vi "kissia_rasPico Module.vi"(5 "Enable":bool=TRUE, 6 "Timeout(s)":dbl=2.0, 7 "Command":T1, 8 "error in (no error)":errorcluster, 10 "VALVE":bool, 11 "VISA resource name":refnum<visa-resource-name>="COM39") -> (0 "error out":errorcluster, 2 "read string":string, 3 "TimeOut":bool, 4 "write string":string)   [LabVIEW 2017]
uses:
  kissia_rasPico Module.ctl
  kissia_ArduinoMicro Module.ctl
  <vilib>/Instr/_visa.llb/VISA Configure Serial Port (Instr).vi
panel:
  out "Bytes at Serial Port":u32
  # "Output Data"
  # "Input Data"
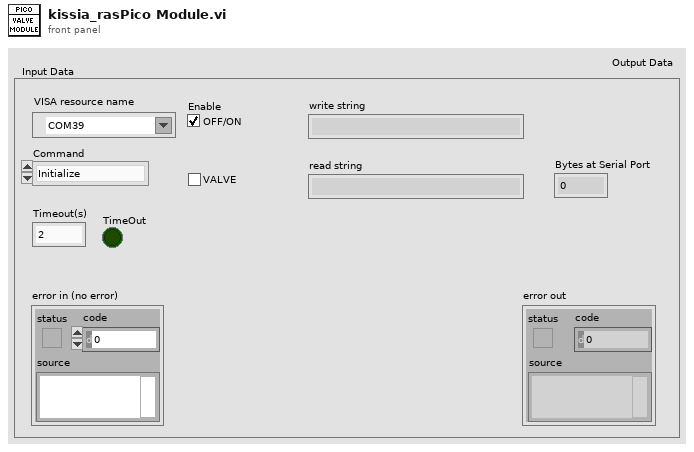
[diagram p1: front panel]
types:
  T1 = typedef "kissia_rasPico Module.ctl" = enum16{"Initialize", "Read Data", "Write Data", "Enable", "Disable", "Shutdown"}
  T2 = typedef "kissia_ArduinoMicro Module.ctl" = enum16{"Initialize", "Read Data", "Write Data", "Enable", "Disable", "Shutdown"}
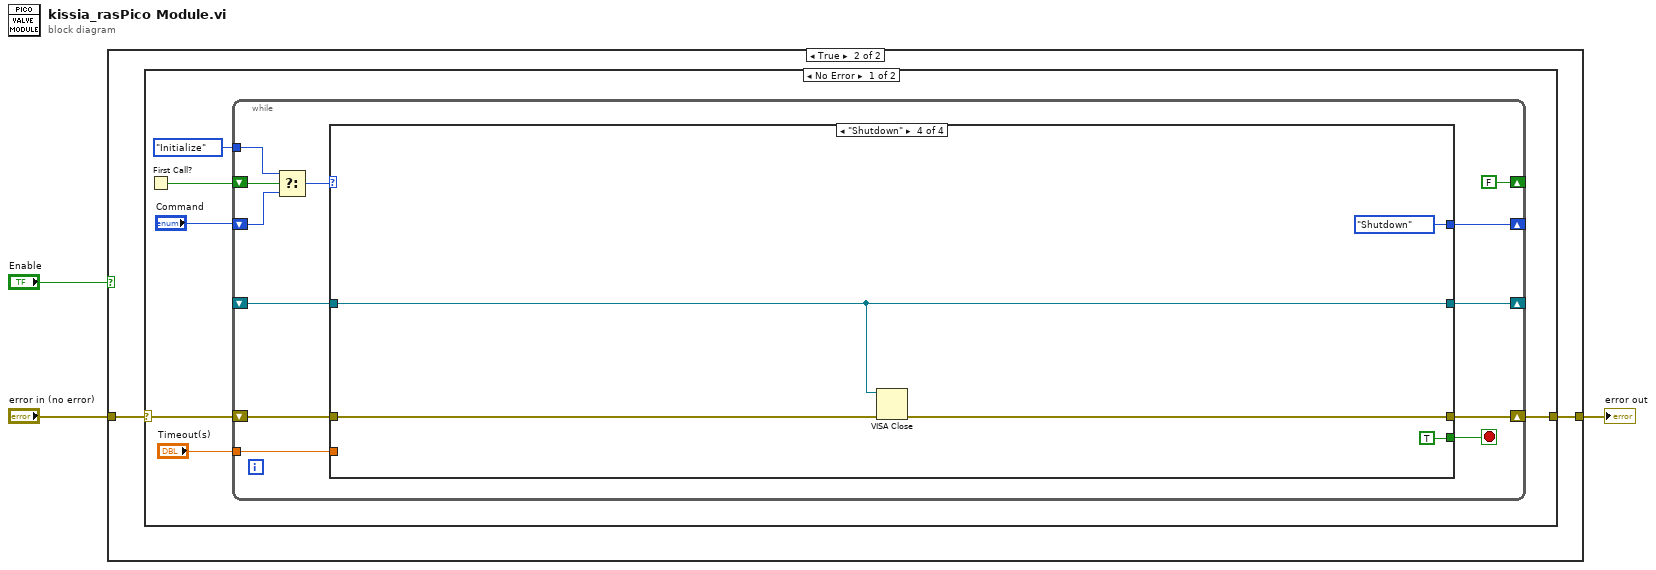
[diagram p0: block diagram]
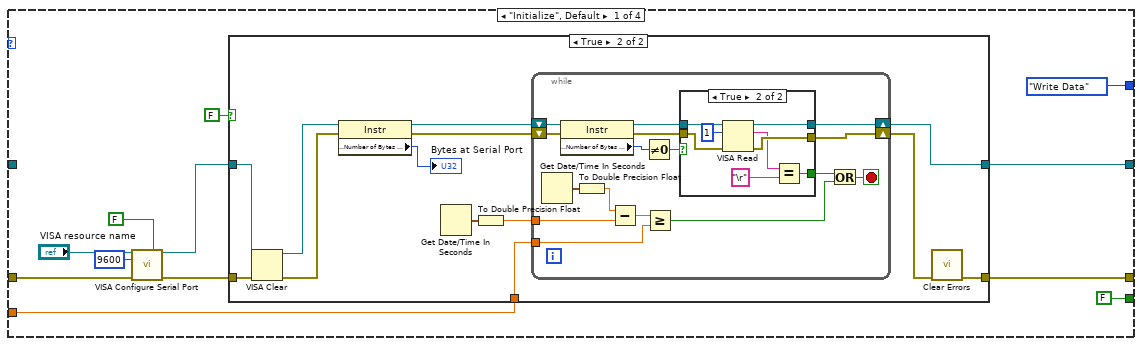
[diagram p3: hidden frame]
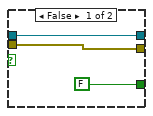
[diagram p5: hidden frame]
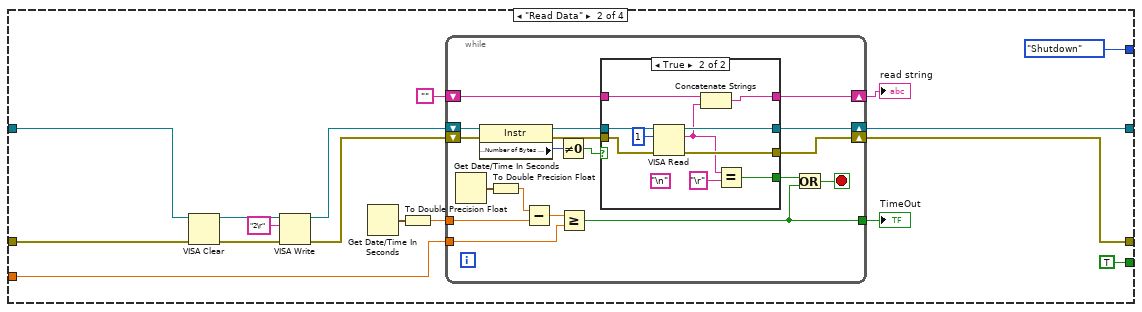
[diagram p6: hidden frame]
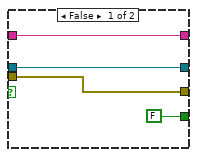
[diagram p7: hidden frame]
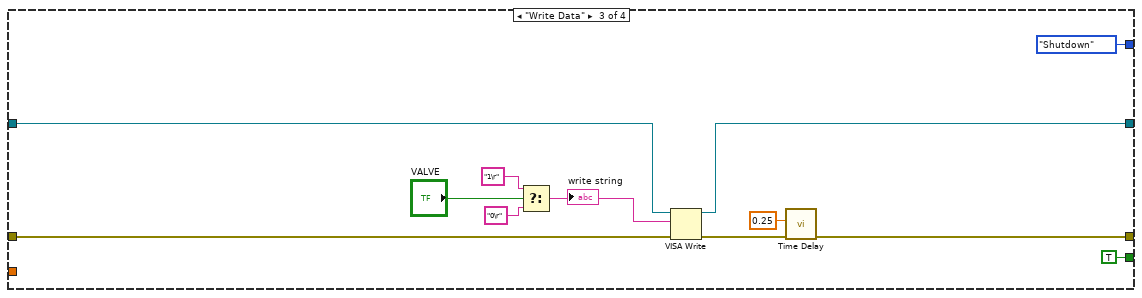
[diagram p8: hidden frame]
diagram:
  n1 = case shown="True" "Enable" {
    tunnel: "error in (no error)" -> [w4 w6]
    tunnel: [w4 w5] -> w2
    frame False {
    }
    frame True {
      n2 = case shown="No Error" w6 {
        selector: w6 -> [w10 w145]
        tunnel: [w9 w145] -> w5
        frame No Error {
          n3 = First Call?() -> (First Call?: T/F=w12:bool)
          n4 = while {
            shift-right: [w15] -> _
            shift-left: "Command" -> [w21]
            shift-right: [w18] -> w9
            shift-left: w10 -> [w19]
            shift-right: [FALSE ("First Call?: T/F")] -> _
            shift-left: w12 -> [w24]
            tunnel: kissia_ArduinoMicro_Module."Initialize" ("t") -> [w23]
            shift-right: [w17] -> _
            shift-left: _ -> [w16]
            tunnel: "Timeout(s)" -> [w13]
            stop <- w14 stop-if-true
            n5 = Select(t=w23, s=w24, f=w21) -> (s? t:f=w20:T2)
            n6 = case shown="\"Shutdown\"" w20 {
              tunnel: w19 -> [w31 w86 w139 w141]
              tunnel: [w26 w87 w133 w140] -> w18
              tunnel: [w30 w88 w136 w142] -> w17
              tunnel: w16 -> [_ w85 w132 w142]
              tunnel: [kissia_ArduinoMicro_Module."Write Data" ("t") kissia_ArduinoMicro_Module."Shutdown" ("t") kissia_ArduinoMicro_Module."Shutdown" ("t") kissia_ArduinoMicro_Module."Shutdown" ("t")] -> w15
              tunnel: [FALSE ("Enable Termination\nChar (T)") TRUE ("Enable Termination\nChar (T)") TRUE ("Enable Termination\nChar (T)") TRUE ("Enable Termination\nChar (T)")] -> w14
              tunnel: w13 -> [w29 w91 _ _]
              frame "Initialize", Default {
                n7 = call-poly "VISA Configure Serial Port"("VISA resource name"="VISA resource name", "Enable Termination\nChar (T)"=FALSE ("Enable Termination\nChar (T)"), "baud rate (9600)"=u32 9600, "error in (no error)"=w31) -> ("VISA resource name out"=w28:refnum<visa-resource-name>, "error out"=w27:errorcluster)  [unwired: 10 in]
                n8 = case shown="True" FALSE {
                  tunnel: [w38 w48] -> w30
                  tunnel: w29 -> [_ w47]
                  tunnel: w28 -> [w38 w46]
                  tunnel: w27 -> [w37 w45]
                  tunnel: [w37 w43] -> w26
                  frame False {
                  }
                  frame True {
                    n9 = VISA Clear(VISA resource name=w46, error in (no error)=w45) -> (VISA resource name out=w40:refnum<visa-resource-name>, error out=w42:errorcluster)
                    n10 = property class="Instr"(reference=w40, error in=w42) -> (reference out=w39:refnum<visa-resource-name>, error out=w41:errorcluster, "Serial Settings:Number of Bytes at Serial Port"=→"Bytes at Serial Port":u32)
                    n11 = Get Date/Time In Seconds() -> (seconds since 1Jan1904=w51:timestamp)
                    n12 = To Double Precision Float(number=w51) -> (double precision float=w50:dbl)
                    n13 = while {
                      tunnel: w50 -> [w52]
                      shift-right: [w62] -> w48
                      shift-left: w39 -> [w60]
                      shift-right: [w61] -> w49
                      shift-left: w41 -> [w59]
                      tunnel: w47 -> [w53]
                      stop <- w67 stop-if-true
                      n14 = Get Date/Time In Seconds() -> (seconds since 1Jan1904=w66:timestamp)
                      n15 = property class="Instr"(reference=w60, error in=w59) -> (reference out=w57:refnum<visa-resource-name>, error out=w58:errorcluster, "Serial Settings:Number of Bytes at Serial Port"=w56:u32)
                      n16 = To Double Precision Float(number=w66) -> (double precision float=w65:dbl)
                      n17 = Subtract(x=w65, y=w52) -> (x-y=w64:dbl)
                      n18 = Not Equal To 0?(x=w56) -> (x != 0?=w55:bool)
                      n19 = Greater Or Equal?(x=w64, y=w53) -> (x >= y?=w63:bool)
                      n20 = case shown="True" w55 {
                        tunnel: [w70 w78] -> w62
                        tunnel: [w69 w77] -> w61
                        tunnel: w58 -> [w69 w76]
                        tunnel: w57 -> [w70 w75]
                        tunnel: [FALSE w72] -> w54
                        frame False {
                        }
                        frame True {
                          n21 = VISA Read(VISA resource name=w75, byte count=u32 1, error in (no error)=w76) -> (VISA resource name out=w78:refnum<visa-resource-name>, read buffer=w73:string, error out=w77:errorcluster)  [unwired: 1 out]
                          n22 = Equal?(x=w73, y="\r" ("Mide")) -> (x = y?=w72:bool)
                        }
                      }
                      n23 = Or(x=w54, y=w63) -> (x .or. y?=w67:bool)
                    }
                    n24 = call <vilib>:"Clear Errors.vi"("error in (no error)"=w49) -> ("error out"=w43:errorcluster)  [unwired: 5 in, 1 out]
                  }
                }
              }
              frame "Read Data" {
                n25 = VISA Clear(VISA resource name=w85, error in (no error)=w86) -> (VISA resource name out=w83:refnum<visa-resource-name>, error out=w81:errorcluster)
                n26 = VISA Write(VISA resource name=w83, write buffer="2\r", error in (no error)=w81) -> (VISA resource name out=w82:refnum<visa-resource-name>, error out=w80:errorcluster)  [unwired: 1 out]
                n27 = Get Date/Time In Seconds() -> (seconds since 1Jan1904=w90:timestamp)
                n28 = To Double Precision Float(number=w90) -> (double precision float=w89:dbl)
                n29 = while {
                  tunnel: w89 -> [w110]
                  shift-right: [w106] -> w88
                  shift-left: w82 -> [w104]
                  shift-right: [w105] -> w87
                  shift-left: w80 -> [w103]
                  tunnel: w91 -> [w108]
                  tunnel: [w107] -> w92
                  shift-right: [w97] -> w84
                  shift-left: "" -> [w98]
                  stop <- w113 stop-if-true
                  n30 = Get Date/Time In Seconds() -> (seconds since 1Jan1904=w112:timestamp)
                  n31 = property class="Instr"(reference=w104, error in=w103) -> (reference out=w101:refnum<visa-resource-name>, error out=w102:errorcluster, "Serial Settings:Number of Bytes at Serial Port"=w100:u32)
                  n32 = To Double Precision Float(number=w112) -> (double precision float=w111:dbl)
                  n33 = Subtract(x=w111, y=w110) -> (x-y=w109:dbl)
                  n34 = Not Equal To 0?(x=w100) -> (x != 0?=w99:bool)
                  n35 = Greater Or Equal?(x=w109, y=w108) -> (x >= y?=w107:bool)
                  n36 = case shown="True" w99 {
                    tunnel: [w117 w127] -> w106
                    tunnel: [w116 w126] -> w105
                    tunnel: w102 -> [w116 w125]
                    tunnel: w101 -> [w117 w124]
                    tunnel: w98 -> [w115 w123]
                    tunnel: [w115 w122] -> w97
                    tunnel: [FALSE w119] -> w96
                    frame False {
                    }
                    frame True {
                      (unwired) "\n"
                      n37 = VISA Read(VISA resource name=w124, byte count=u32 1, error in (no error)=w125) -> (VISA resource name out=w127:refnum<visa-resource-name>, read buffer=w120:string, error out=w126:errorcluster)  [unwired: 1 out]
                      n38 = Concatenate Strings(w123, w120) -> (w122:string)
                      n39 = Equal?(x=w120, y="\r" ("Mide")) -> (x = y?=w119:bool)
                    }
                  }
                  n40 = Or(x=w96, y=w107) -> (x .or. y?=w113:bool)
                }
                "read string" <- w84
                "TimeOut" <- w92
              }
              frame "Write Data" {
                n41 = Select(t="1\r" ("write buffer"), s="VALVE", f="0\r" ("write buffer")) -> (s? t:f=w128:string)
                "write string" <- w128
                n42 = VISA Write(VISA resource name=w132, write buffer=w128, error in (no error)=w139) -> (VISA resource name out=w136:refnum<visa-resource-name>, error out=w134:errorcluster)  [unwired: 1 out]
                n43 = call "Time Delay"("error in (no error)"=w134, "Delay Time (s)"=0.25) -> ("error out"=w133:errorcluster)  [unwired: 9 in]
              }
              frame "Shutdown" {
                n44 = VISA Close(VISA resource name=w142, error in (no error)=w141) -> (error out=w140:errorcluster)
              }
            }
          }
        }
        frame Error {
        }
      }
    }
  }
  "error out" <- w2
